vi "Keithley Sweep and Acquire Measurements_averaging.vi"(6 "Scan Settings JV":T1={"Light intensity (Suns)"=1.0, "Pre-bias time (s)"=0.0, "Maximum voltage (V)"=0.0, "Minimum voltage (V)"=-1.4, "Range Options"=4, "1st scan FB to SC?"=TRUE, "Step Size (V)"=0.01, "Source Delay (s)"=0.01, "Inverted device"=FALSE, "Measure stabilized power output"=TRUE, "Stabilzation time (s)"=40.0, "Use Vmp from JV scan"=TRUE, "Stabization voltage (V)"=0.8, "Only stabilize best pixels"=TRUE, "Number of pixels to stabilize \nper substrate"=0, "Stabilization time step (s)"=1.0, "Use max power tracking"=FALSE, "Pre-bias voltage (V)"=-1.4, "No. of data point averages"=1.0, "No. of J-V averages"=1.0, "Integration time (ms)"=200.0} {"Number of pixels to stabilize \nper substrate" items=["1", "2", "3", "4", "5", "6", "7", "8"]; "Range Options" items=["Auto Range", "100 uA", "1 mA", "10 mA", "100 mA", "1A"]}, 7 "Sweep Direction":u16(ring) items=["Low to high", "High to low"], 11 "VISA resource name":refnum<visa-resource-name>) -> (2 "Data Array":dbl[][](array[numeric]), 3 "VISA resource name out":refnum<visa-resource-name>)   [LabVIEW 2011]
doc: "Configures a sweep and takes voltage and current readings at each point."
uses:
  Typedefs/Scan settings.ctl
  <instrlib>/keithley_24xx/Keithley 24XX/Public/Data/Read (Multiple Points).vi
  <instrlib>/keithley_24xx/Keithley 24XX/Keithley 24XX.lvlib
panel:
  in  "Manual Range (1.0)":dbl=1.0
  in  "Source Mode  (0: Voltage)":u16(ring) items=["Voltage", "Current"]
  in  "Compliance  Level":dbl=0.1
  # "(c) 2006 National Instruments.  ALL RIGHTS RESERVED."
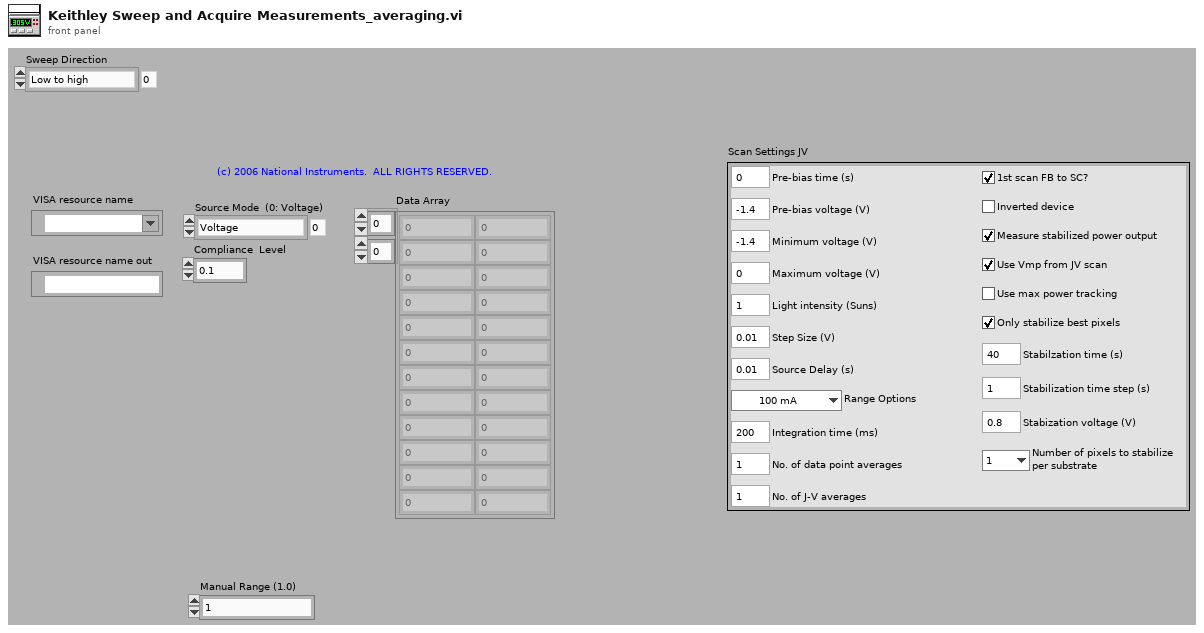
[diagram p1: front panel]
types:
  T1 = typedef "Scan settings.ctl" = cluster{"Light intensity (Suns)":dbl, "Pre-bias time (s)":dbl, "Maximum voltage (V)":dbl, "Minimum voltage (V)":dbl, "Range Options":u16, "1st scan FB to SC?":bool, "Step Size (V)":dbl, "Source Delay (s)":dbl, "Inverted device":bool, "Measure stabilized power output":bool, "Stabilzation time (s)":dbl, "Use Vmp from JV scan":bool, "Stabization voltage (V)":dbl, "Only stabilize best pixels":bool, "Number of pixels to stabilize \nper substrate":u16, "Stabilization time step (s)":dbl, "Use max power tracking":bool, "Pre-bias voltage (V)":dbl, "No. of data point averages":dbl, "No. of J-V averages":dbl, "Integration time (ms)":dbl}
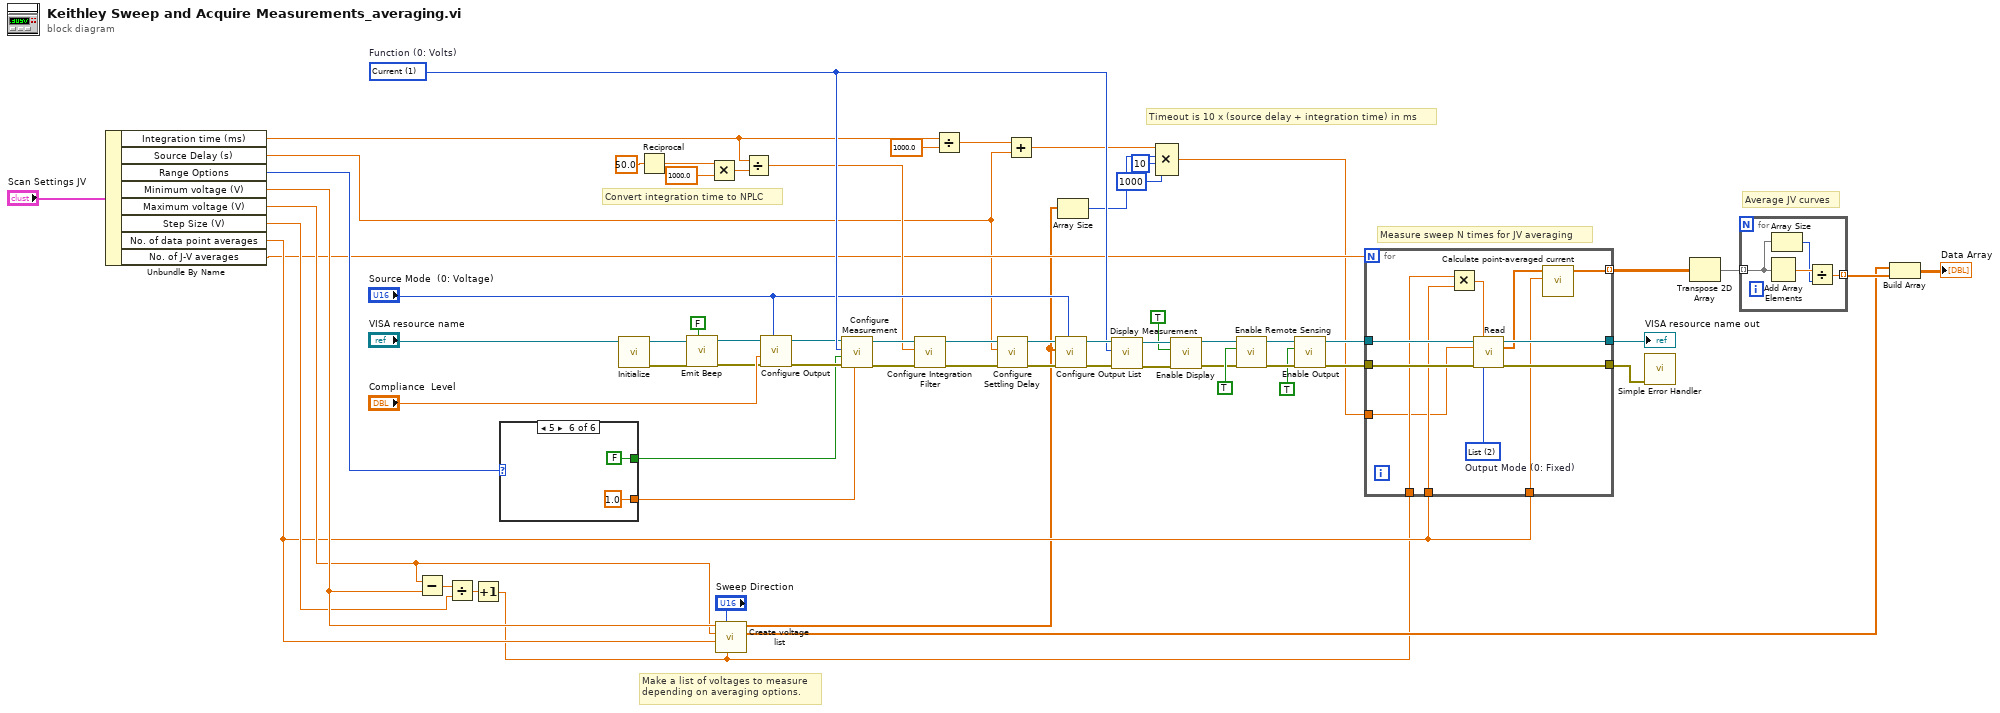
[diagram p0: block diagram]
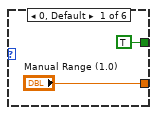
[diagram p2: hidden frame]
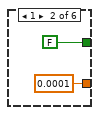
[diagram p3: hidden frame]
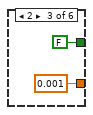
[diagram p4: hidden frame]
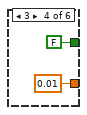
[diagram p5: hidden frame]
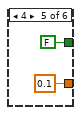
[diagram p6: hidden frame]
diagram:
  w51 = u16 1 items=["Volts", "Current", "Resistance"]  # Function (0: Volts)
  # "Average JV curves"
  # "Measure sweep N times for JV averaging"
  # "Convert integration time to NPLC"
  # "Timeout is 10 x (source delay + integration time) in ms"
  # "Make a list of voltages to measure\ndepending on averaging options."
  n1 = Unbundle By Name("Scan Settings JV") -> ("Integration time (ms)"=w3:dbl, "Source Delay (s)"=w9:dbl, "Range Options"=w17:u16, "Minimum voltage (V)"=w16:dbl, "Maximum voltage (V)"=w15:dbl, "Step Size (V)"=w14:dbl, "No. of data point averages"=w13:dbl, "No. of J-V averages"=w11:dbl)
  n2 = Subtract(x=w15, y=w16) -> (x-y=w20:dbl)
  n3 = Divide(x=w20, y=w14) -> (x/y=w19:dbl)
  n4 = Increment(x=w19) -> (x+1=w12:dbl)
  n5 = case shown="5" w17 {
    tunnel: ["Manual Range (1.0)" 0.0001 ("Manual Range (1.0)") 0.001 ("Manual Range (1.0)") 0.01 ("Manual Range (1.0)") 0.1 ("Manual Range (1.0)") 1.0 ("Manual Range (1.0)")] -> w24
    tunnel: [TRUE FALSE FALSE FALSE FALSE FALSE] -> w23
    frame 0, Default {
    }
    frame 1 {
    }
    frame 2 {
    }
    frame 3 {
    }
    frame 4 {
    }
    frame 5 {
    }
  }
  n6 = call <instrlib>:"Initialize.vi"("VISA resource name"="VISA resource name") -> ("error out"=w46:errorcluster, "VISA resource name out"=w47:refnum<visa-resource-name>)  [unwired: 9 in]
  n7 = Reciprocal(x=50.0) -> (1/x=w30:dbl)
  n8 = call <instrlib>:"Emit Beep.vi"("Enable Beep (F)"=FALSE, "error in (no error)"=w46, "VISA resource name"=w47) -> ("error out"=w39:errorcluster, "VISA resource name out"=w40:refnum<visa-resource-name>)  [unwired: 7 in]
  n9 = Multiply(x=w30, y=1000.0) -> (x*y=w29:dbl)
  n10 = call "Create voltage list.vi"("No. of measurement points"=w12, "Sweep Direction"="Sweep Direction", "No. of data point averages"=w13, "Maximum voltage (V)"=w15, "Minimum voltage (V)"=w16) -> ("Voltages"=w22:dbl[], "Voltage list for measurement"=w10:dbl[])  [unwired: 5 in]
  n11 = Divide(x=w3, y=w29) -> (x/y=w28:dbl)
  n12 = call <instrlib>:"Configure Output.vi"("Source Mode  (0: Voltage)"="Source Mode  (0: Voltage)", "error in (no error)"=w39, "Compliance  Level (0.1)"="Compliance  Level", "VISA resource name"=w40) -> ("error out"=w35:errorcluster, "VISA resource name out"=w36:refnum<visa-resource-name>)  [unwired: 6 in]
  n13 = call <instrlib>:"Configure Measurement.vi"("Manual Range (1.0)"=w24, "error in (no error)"=w35, "Enable Auto Range (T:Enable)"=w23, "Function (0: Volts)"=w51, "VISA resource name"=w36) -> ("error out"=w54:errorcluster, "VISA resource name out"=w55:refnum<visa-resource-name>)  [unwired: 5 in]
  n14 = call <instrlib>:"Configure Integration Filter.vi"("error in (no error)"=w54, "Measurement Speed (1 PLC)"=w28, "VISA resource name"=w55) -> ("error out"=w33:errorcluster, "VISA resource name out"=w34:refnum<visa-resource-name>)  [unwired: 7 in]
  n15 = Divide(x=w3, y=1000.0) -> (x/y=w1:dbl)
  n16 = call <instrlib>:"Configure Settling Delay.vi"("error in (no error)"=w33, "Manual Settling Delay (0 sec)"=w9, "VISA resource name"=w34) -> ("error out"=w48:errorcluster, "VISA resource name out"=w49:refnum<visa-resource-name>)  [unwired: 7 in]
  n17 = Add(x=w1, y=w9) -> (x+y=w8:dbl)
  n18 = call <instrlib>:"Configure Output List.vi"("Source Mode  (0: Voltage)"="Source Mode  (0: Voltage)", "error in (no error)"=w48, "Output List"=w10, "VISA resource name"=w49) -> ("error out"=w52:errorcluster, "VISA resource name out"=w53:refnum<visa-resource-name>)  [unwired: 6 in]
  n19 = Array Size(array=w10) -> (size(s)=w7:i32)
  n20 = call <instrlib>:"Display Measurement.vi"("error in (no error)"=w52, "Displayed Measurement (0: Voltage)"=w51, "VISA resource name"=w53) -> ("error out"=w44:errorcluster, "VISA resource name out"=w45:refnum<visa-resource-name>)  [unwired: 7 in]
  n21 = Compound Arithmetic op=MULTIPLY(w8, w7, 10 ("value"), 1000 ("value")) -> (w5:dbl)
  n22 = call <instrlib>:"Enable Display.vi"("error in (no error)"=w44, "Enable Display (T: Enable)"=TRUE, "VISA resource name"=w45) -> ("error out"=w42:errorcluster, "VISA resource name out"=w43:refnum<visa-resource-name>)  [unwired: 7 in]
  n23 = call <instrlib>:"Enable Remote Sensing.vi"("error in (no error)"=w42, "Enable Remote Sensing (T: Enable)"=TRUE ("Enable Output (T: Enable)"), "VISA resource name"=w43) -> ("error out"=w59:errorcluster, "VISA resource name out"=w60:refnum<visa-resource-name>)  [unwired: 7 in]
  n24 = call <instrlib>:"Enable Output.vi"("error in (no error)"=w59, "Enable Output (T: Enable)"=TRUE, "VISA resource name"=w60) -> ("error out"=w64:errorcluster, "VISA resource name out"=w63:refnum<visa-resource-name>)  [unwired: 7 in]
  n25 = for {
    N: w11 -> [_]
    tunnel: w64 -> [w88]
    tunnel: w63 -> [w87]
    tunnel: [w86] -> w62
    tunnel: [w85] -> w61
    tunnel: w13 -> [w82]
    tunnel: [w81] -> w27 mode=indexing
    tunnel: w13 -> [w80]
    tunnel: w12 -> [w79]
    tunnel: w5 -> [w78]
    w89 = u16 2 items=["Fixed", "Sweep", "List"]  # Output Mode (0: Fixed)
    n26 = Multiply(x=w79, y=w80) -> (x*y=w84:dbl)
    n27 = call-poly <instrlib>:"Read.vi"("VISA resource name"=w87, "Sample Count (1)"=w84, "Timeout (10000 ms)"=w78, "error in (no error)"=w88, "Output Mode (0: Fixed)"=w89) -> ("VISA resource name out"=w85:refnum<visa-resource-name>, "Current"=w83:sgl[], "error out"=w86:errorcluster)  [unwired: 4 in, 4 out]
    n28 = call "Calculate point-averaged current.vi"("No. of data point averages"=w82, "Current list"=w83) -> ("Point-averaged current"=w81:sgl[])  [unwired: 9 in]
  }
  "VISA resource name out" <- w61
  n29 = call <vilib>:"Simple Error Handler.vi"("error in (no error)"=w62) -> ()  [unwired: 4 in, 5 out]
  n30 = Transpose 2D Array(2D array=w27) -> (transposed array=w25:sgl[][])
  n31 = for {
    tunnel: w25 -> [w92] mode=indexing
    tunnel: [w90] -> w26 mode=indexing
    n32 = Add Array Elements(numeric array=w92) -> (sum=w93:sgl)
    n33 = Array Size(array=w92) -> (size(s)=w91:i32)
    n34 = Divide(x=w93, y=w91) -> (x/y=w90:sgl)
  }
  n35 = Build Array(w22, w26) -> (→"Data Array":dbl[][])
